vi "Find Average Center.vi"(4 "Position":i32, 5 "Tray Number":i32, 7 "XYZTheta":dbl[](array[numeric]), 8 "Gantry 2":refnum<k24>) -> (1 "XYZTheta":dbl[](array[numeric]), 2 "Gantry 3":refnum<k24>)   [LabVIEW 2020, in "Component Tray.lvclass"]
uses:
  Component Tray.lvclass
  Find Component.ctl
  C:/Program Files (x86)/Aerotech/A3200/LabVIEW/2010/Bin/Aerotech.A3200.dll
  Program Files (x86)/Aerotech/A3200/LabVIEW/2010/Bin/Aerotech.A3200.dll
  Controller/Camera/Machine Vision.ctl
  Controller/Motion/Motion.lvclass
  Controller/Motion/A3200/A3200.lvclass
  Controller/Camera/Camera.lvclass
panel:
  in  "?":bool
  out "Image":T1(plugin-control)
  out "Camera":dbl[](array[numeric])
  in  "Machine Vision":T2
  out "Gantry":dbl[](array[numeric])
  out "Sum":dbl[](array[numeric])
  out "BR XY":dbl[](array[numeric])
  out "TR XY":dbl[](array[numeric])
  out "BL XY":dbl[](array[numeric])
  out "TL XY":dbl[](array[numeric])
  in  "Record Top Right":bool
  in  "Record Bottom Right":bool
  in  "Record Bottom Left":bool
  in  "Record Top Left":bool
  in  "Go to Bottom Right":bool
  in  "Go to Top Right":bool
  in  "Go to Bottom Left":bool
  in  "Go to Top Left":bool
  in  "Joystick":bool
  in  "Go to Center":bool
  in  "Component":T3
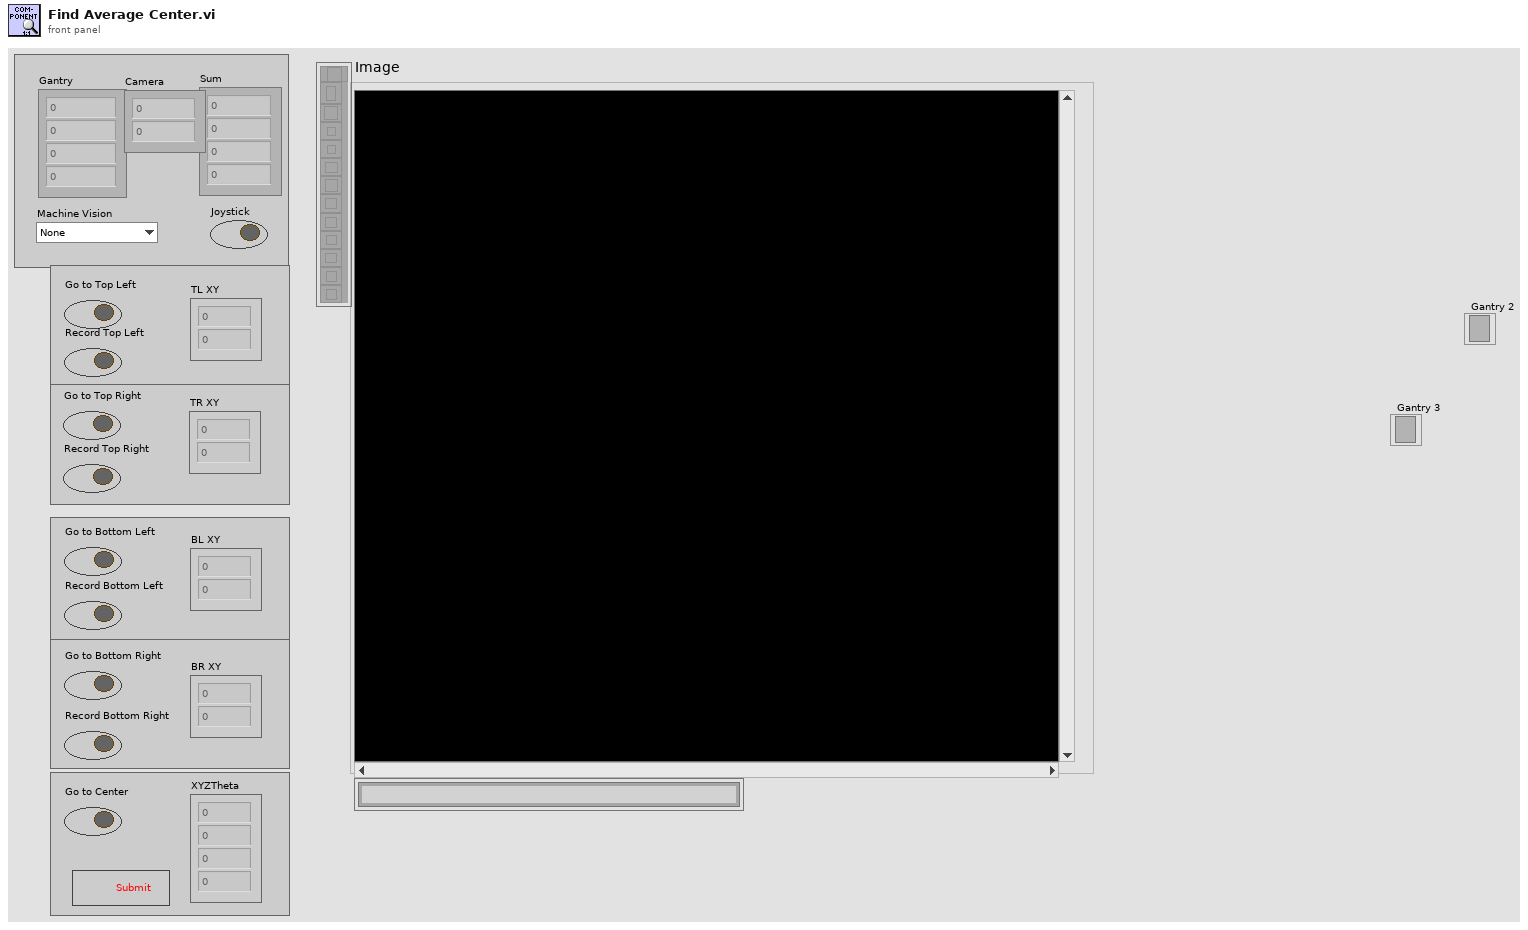
[diagram p1: front panel]
types:
  T1 = typedef "IMAQ Image.ctl" = refnum<image>
  T2 = typedef "Camera.lvclass/Machine Vision.ctl" = enum16{"None", "Tray Fiducials", "HPK Silicon", "Hexaboard", "Corner (TL, BR)", "Corner (BL, TR)"}
  T3 = typedef "Component Tray.lvclass/Find Component.ctl" = cluster{"New Fiducials":dbl[], "Past Fiducials":dbl[], "XYZTheta":dbl[], "Fiducials Path":path, "Position":i32}
  T4 = typedef "File Paths.ctl" = cluster{"Glue Pattern Folder":path, "Carrier Tray Folder":path, "Pick Up Tool Fixture Folder":path, "Components Folder":path, "Bellows Tool Offset.txt":path, "Pick Up Tool Offset.txt":path, "Dispense Tip Offset.txt":path, "Log Files":path}
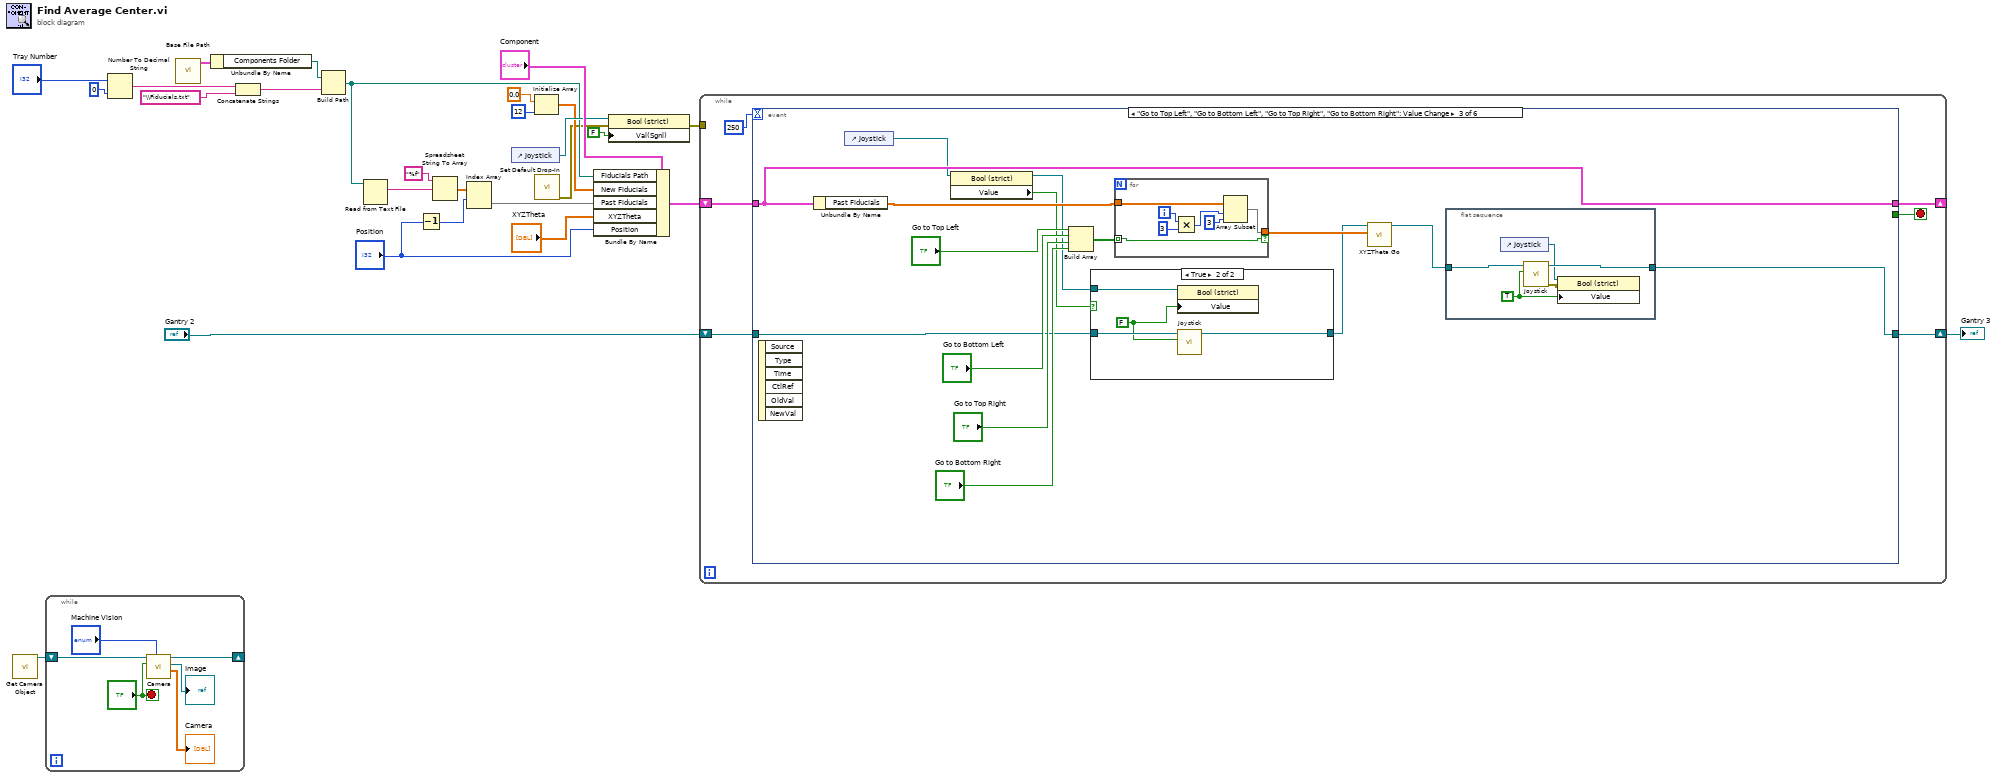
[diagram p0: block diagram]
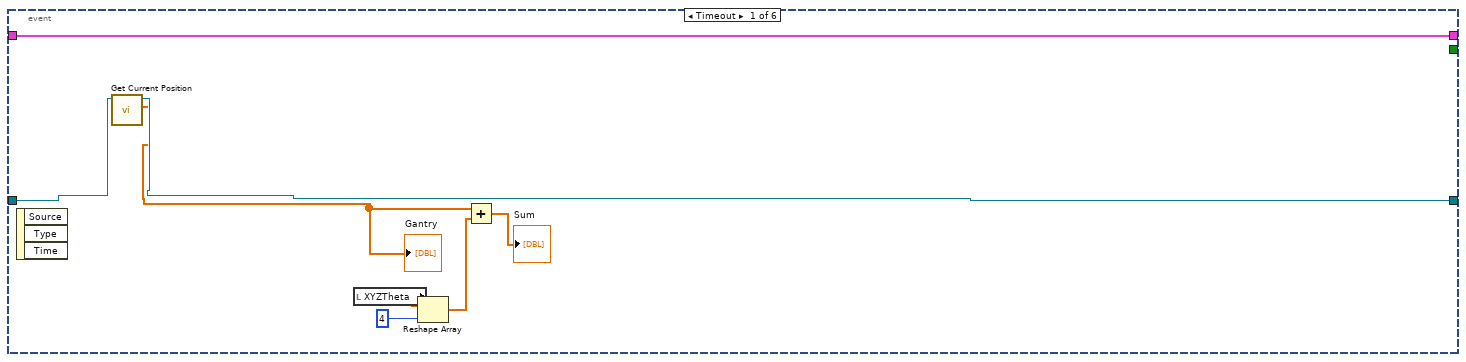
[diagram p2: hidden frame]
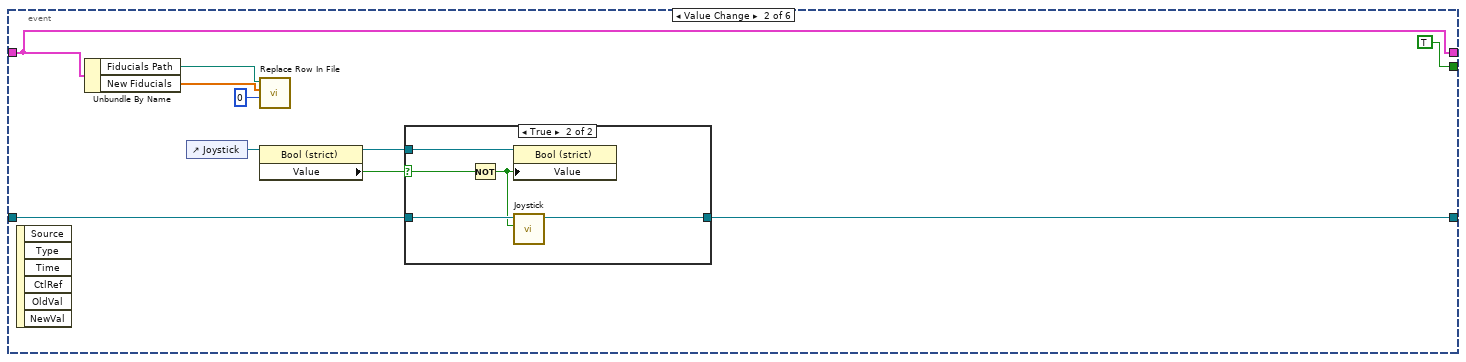
[diagram p3: hidden frame]
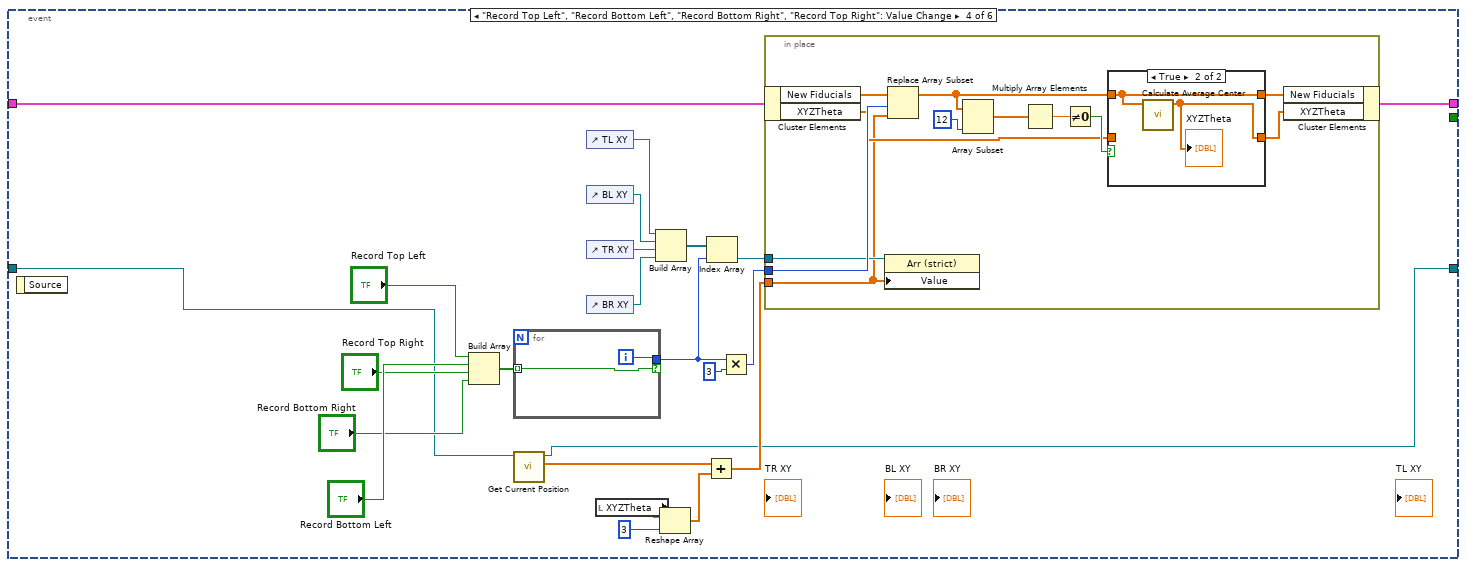
[diagram p6: hidden frame]
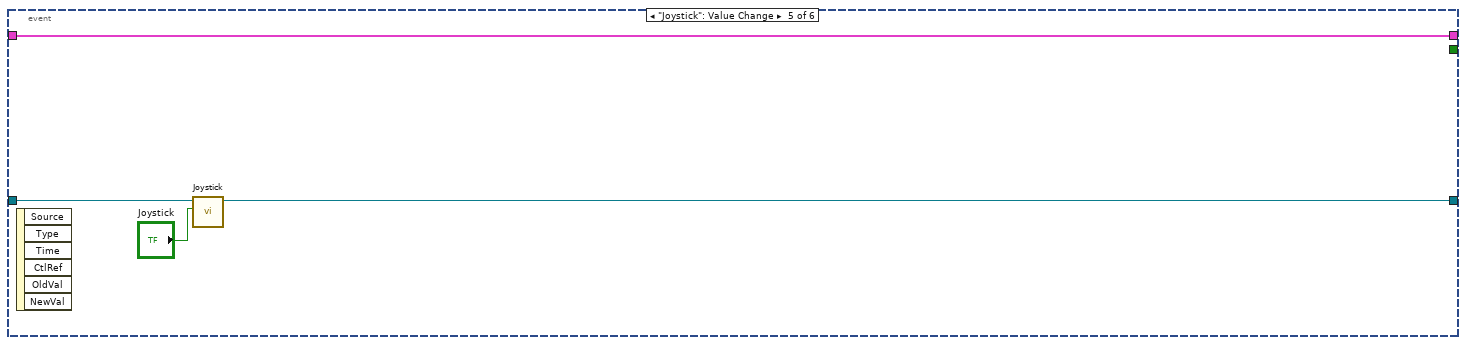
[diagram p8: hidden frame]
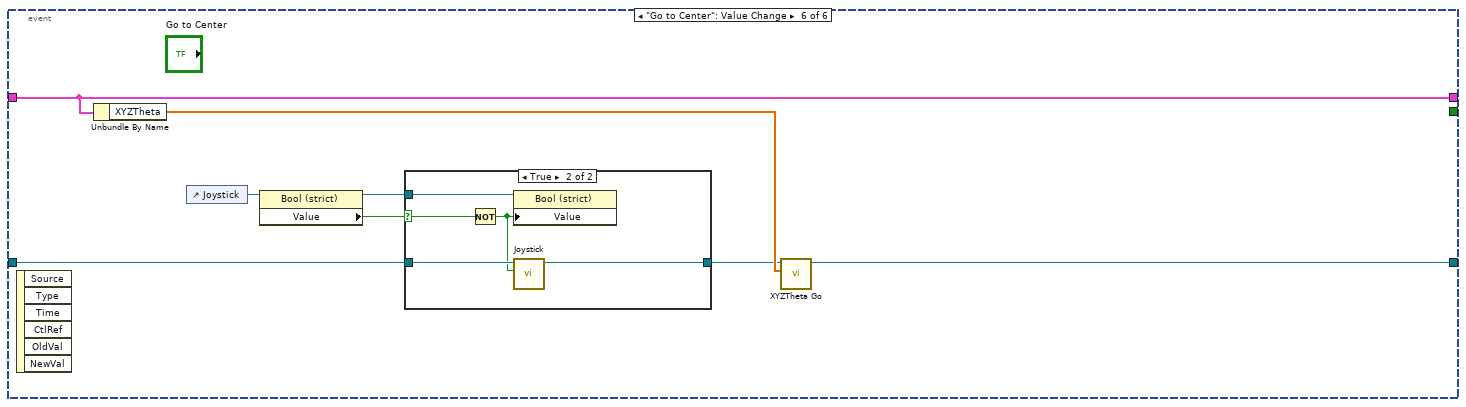
[diagram p9: hidden frame]
diagram:
  n1 = call "Get Camera Object.vi"() -> ("Camera out"=w2:refnum<class "Camera.lvclass">)  [unwired: 10 in, 1 out]
  n2 = while {
    shift-right: [w32] -> _
    shift-left: w2 -> [w33]
    stop <- "?" stop-if-true
    n3 = call "Camera.vi"("Machine Vision"="Machine Vision", "Stop"="?", "Camera in"=w33) -> ("Camera"=→"Camera":dbl[], "Image"=→"Image":T1, "Camera out"=w32:refnum<class "Camera.lvclass">)  [unwired: 5 in, 1 out]
  }
  n4 = Number To Decimal String(number="Tray Number", width (-)=i16 0) -> (decimal integer string=w17:string)
  n5 = call "Base File Path.vi"() -> ("Paths Out"=w14:T4)  [unwired: 11 in]
  n6 = Unbundle By Name(w14) -> ("Components Folder"=w16:path)
  n7 = Concatenate Strings(w17, "\\Fiducials.txt" ("string")) -> (w19:string)
  n8 = Build Path(base path=w16, name or relative path=w19) -> (appended path=w8:path)
  n9 = Read from Text File(file (use dialog)=w8) -> (text=w20:string)  [unwired: 3 in, 3 out]
  n10 = Decrement(x="Position") -> (x-1=w5:i32)
  n11 = Spreadsheet String To Array(format string="%f", spreadsheet string=w20) -> (array=w22:dbl[][])  [unwired: 2 in]
  n12 = Index Array(array=w22, index (row)=w5) -> (element=w12:dbl[])  [unwired: 1 in]
  n13 = control-ref of="Joystick"() -> (w25:refnum<vi>)
  n14 = Initialize Array(0.0 ("element"), 12 ("dimension size")) -> (w11:dbl[])
  n15 = call "Set Default Drop-In.vi"() -> ("error out"=w4:errorcluster)  [unwired: 11 in]
  n16 = Bundle By Name(cluster="Component", "Fiducials Path"=w8, "New Fiducials"=w11, "Past Fiducials"=w12, "XYZTheta"="XYZTheta", "Position"="Position") -> (w26:T3)
  n17 = property class="Bool (strict)"(reference=w25, error in=w4, "Val(Sgnl)"=FALSE) -> (error out=w23:errorcluster)  [unwired: 1 out]
  n18 = while {
    shift-right: [w37] -> _
    shift-left: w26 -> [w38]
    tunnel: w23 -> [_]
    shift-right: [w34] -> w3
    shift-left: "Gantry 2" -> [w35]
    stop <- w39 stop-if-true
    n19 = event shown="[2] \"Go to Top Left\", \"Go to Bottom Left\", \"Go to Top Right\", \"Go to Bottom Right\": Value Change" {
      selector: _ -> [_ _ _ _ _ _]
      dyn-events: _ -> [_ _ _ _ _ _]
      timeout: 250 -> [_ _ _ _ _ _]
      tunnel: [_ TRUE _ _ _ _] -> w39
      tunnel: w38 -> [w46 w49 w71 w118 w140 w147]
      tunnel: [w46 w49 w71 w117 w140 w147] -> w37
      tunnel: w35 -> [w42 w53 w67 w97 w139 w142]
      tunnel: [w41 w52 w64 w96 w137 w143] -> w34
      event Timeout {
        n20 = event-data() -> ()  [unwired: 1 in, 3 out]
        n21 = call "Get Current Position.vi"("Gantry 2"=w42) -> ("XYZTheta Out"=w40:dbl[], "Gantry 3"=w41:refnum<k24>)  [unwired: 8 in, 1 out]
        "Gantry" <- w40
        n22 = local read "XYZTheta"() -> (w45:dbl[])
        n23 = Reshape Array(w45, 4 ("dimension size")) -> (w43:dbl[])
        n24 = Add(x=w40, y=w43) -> (x+y=→"Sum":dbl[])
      }
      event Value Change {
        n25 = event-data() -> ()  [unwired: 1 in, 6 out]
        n26 = Unbundle By Name(w49) -> ("Fiducials Path"=w51:path, "New Fiducials"=w50:dbl[])
        n27 = control-ref of="Joystick"() -> (w54:refnum<vi>)
        n28 = call "Replace Row In File.vi"("Index"=0, "Insert Array"=w50, "Path"=w51) -> ()  [unwired: 8 in, 1 out]
        n29 = property class="Bool (strict)"(reference=w54) -> (reference out=w55:refnum<vi>, "Value"=w56:bool)  [unwired: 1 in, 1 out]
        n30 = case shown="True" w56 {
          selector: w56 -> [_ w63]
          tunnel: w55 -> [_ w62]
          tunnel: w53 -> [w58 w61]
          tunnel: [w58 w59] -> w52
          frame False {
          }
          frame True {
            n31 = Not(x=w63) -> (.not. x?=w60:bool)
            n32 = property class="Bool (strict)"(reference=w62, "Value"=w60) -> ()  [unwired: 1 in, 2 out]
            n33 = call "Joystick.vi"("Joystick"=w60, "Gantry 2"=w61) -> ("Gantry 3"=w59:refnum<k24>)  [unwired: 8 in, 1 out]
          }
        }
      }
      event "Go to Top Left", "Go to Bottom Left", "Go to Top Right", "Go to Bottom Right": Value Change {
        n34 = event-data() -> ()  [unwired: 1 in, 6 out]
        n35 = Unbundle By Name(w71) -> ("Past Fiducials"=w73:dbl[])
        n36 = control-ref of="Joystick"() -> (w68:refnum<vi>)
        n37 = property class="Bool (strict)"(reference=w68) -> (reference out=w69:refnum<vi>, "Value"=w70:bool)  [unwired: 1 in, 1 out]
        n38 = Build Array("Go to Top Left", "Go to Bottom Left", "Go to Top Right", "Go to Bottom Right") -> (w74:bool[])
        n39 = case shown="True" w70 {
          tunnel: w69 -> [_ w88]
          tunnel: w67 -> [w84 w87]
          tunnel: [w84 w86] -> w66
          frame False {
          }
          frame True {
            w85 = FALSE
            n40 = property class="Bool (strict)"(reference=w88, "Value"=w85) -> ()  [unwired: 1 in, 2 out]
            n41 = call "Joystick.vi"("Joystick"=w85, "Gantry 2"=w87) -> ("Gantry 3"=w86:refnum<k24>)  [unwired: 8 in, 1 out]
          }
        }
        n42 = for {
          tunnel: w74 -> [w95] mode=indexing
          tunnel: w73 -> [w94]
          tunnel: [w89] -> w72 if=w95
          i -> [w92]
          n43 = Multiply(x=w92, y=3) -> (x*y=w90:i32)
          n44 = Array Subset(array=w94, index=w90, length=3) -> (w89:dbl[])
        }
        n45 = call "XYZTheta Go.vi"("XYZTheta In"=w72, "Gantry 2"=w66) -> ("Gantry 3"=w65:refnum<k24>)  [unwired: 7 in, 2 out]
        n46 = flat-sequence {
          tunnel: [w81] -> w64
          tunnel: w65 -> [w79]
          frame #0 {
            w83 = TRUE
            n47 = control-ref of="Joystick"() -> (w80:refnum<vi>)
            n48 = call "Joystick.vi"("Joystick"=w83, "Gantry 2"=w79) -> ("error out"=w82:errorcluster, "Gantry 3"=w81:refnum<k24>)  [unwired: 8 in]
            n49 = property class="Bool (strict)"(reference=w80, error in=w82, "Value"=w83) -> ()  [unwired: 2 out]
          }
        }
      }
      event "Record Top Left", "Record Bottom Left", "Record Bottom Right", "Record Top Right": Value Change {
        n50 = event-data() -> ()  [unwired: 1 in, 1 out]
        n51 = Build Array("Record Top Left", "Record Bottom Left", "Record Top Right", "Record Bottom Right") -> (w112:bool[])
        n52 = for {
          tunnel: w112 -> [w119] mode=indexing
          tunnel: [w120] -> w104 if=w119
          i -> [w120]
        }
        n53 = call "Get Current Position.vi"("Gantry 2"=w97) -> ("XYZTheta Out"=w98:dbl[], "Gantry 3"=w96:refnum<k24>)  [unwired: 8 in, 1 out]
        n54 = control-ref of="TL XY"() -> (w111:refnum<vi>)
        n55 = control-ref of="BL XY"() -> (w110:refnum<vi>)
        n56 = control-ref of="TR XY"() -> (w109:refnum<vi>)
        n57 = control-ref of="BR XY"() -> (w108:refnum<vi>)
        n58 = local read "XYZTheta"() -> (w101:dbl[])
        n59 = Build Array(w111, w110, w109, w108) -> (w107:refnum<vi>[])
        n60 = Reshape Array(w101, 3 ("dimension size")) -> (w100:dbl[])
        n61 = Add(x=w98, y=w100) -> (x+y=w99:dbl[])
        n62 = Index Array(array=w107, index=w104) -> (element=w106:refnum<vi>)
        n63 = Multiply(x=w104, y=3) -> (x*y=w102:i32)
        n64 = in-place {
          in-place-border: w102 -> [w130]
          in-place-border: w106 -> [w127]
          in-place-border: w99 -> [w125]
          n65 = in-place-cluster #1(w118) -> ("New Fiducials"=w131:dbl[], "XYZTheta"=w126:dbl[])
          n66 = property class="Arr (strict)"(reference=w127, "Value"=w125) -> ()  [unwired: 1 in, 2 out]
          n67 = Replace Array Subset(array=w131, new element=w125, index=w130) -> (w124:dbl[])
          n68 = Array Subset(array=w124, length=12) -> (w122:dbl[])  [unwired: 1 in]
          n69 = Multiply Array Elements(1:w122) -> (0:w121:dbl)
          n70 = Not Equal To 0?(x=w121) -> (x != 0?=w128:bool)
          n71 = case shown="True" w128 {
            tunnel: [w133 w135] -> w132
            tunnel: w124 -> [w134 w136]
            tunnel: [w134 w136] -> w129
            tunnel: w126 -> [w133 _]
            frame False {
            }
            frame True {
              n72 = call "Calculate Average Center.vi"("Gantry Fiducials"=w136) -> ("XYZTheta"=w135:dbl[])  [unwired: 10 in]
              "XYZTheta" <- w135
            }
          }
          n73 = in-place-cluster #1("New Fiducials"=w129, "XYZTheta"=w132) -> (w117:T3)
        }
      }
      event "Joystick": Value Change {
        n74 = event-data() -> ()  [unwired: 1 in, 6 out]
        n75 = call "Joystick.vi"("Joystick"="Joystick", "Gantry 2"=w139) -> ("Gantry 3"=w137:refnum<k24>)  [unwired: 8 in, 1 out]
      }
      event "Go to Center": Value Change {
        n76 = event-data() -> ()  [unwired: 1 in, 6 out]
        n77 = Unbundle By Name(w147) -> ("XYZTheta"=w148:dbl[])
        n78 = control-ref of="Joystick"() -> (w144:refnum<vi>)
        n79 = property class="Bool (strict)"(reference=w144) -> (reference out=w145:refnum<vi>, "Value"=w146:bool)  [unwired: 1 in, 1 out]
        n80 = case shown="True" w146 {
          selector: w146 -> [_ w154]
          tunnel: w145 -> [_ w153]
          tunnel: w142 -> [w149 w152]
          tunnel: [w149 w151] -> w141
          frame False {
          }
          frame True {
            n81 = Not(x=w154) -> (.not. x?=w150:bool)
            n82 = property class="Bool (strict)"(reference=w153, "Value"=w150) -> ()  [unwired: 1 in, 2 out]
            n83 = call "Joystick.vi"("Joystick"=w150, "Gantry 2"=w152) -> ("Gantry 3"=w151:refnum<k24>)  [unwired: 8 in, 1 out]
          }
        }
        n84 = call "XYZTheta Go.vi"("XYZTheta In"=w148, "Gantry 2"=w141) -> ("Gantry 3"=w143:refnum<k24>)  [unwired: 7 in, 2 out]
      }
    }
  }
  "Gantry 3" <- w3
